vi "ARC_Queue Valid.vi"(8 "error in (no error)":errorcluster caption="Error In (no error)", 11 "Queue Name(unamed)":string) -> (0 "error out":errorcluster caption="Error Out", 2 "Not Exist?":bool, 3 "Empty Queue Name?":bool)   [LabVIEW 2016]
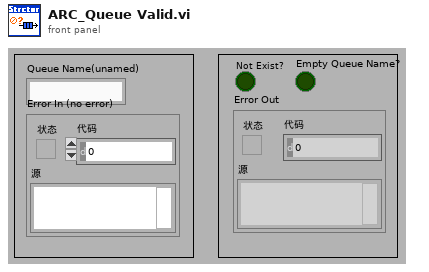
[diagram p1: front panel]
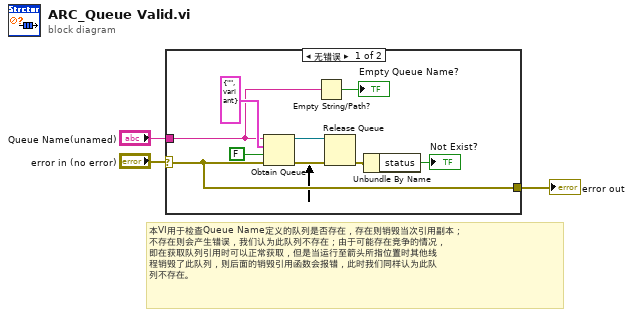
[diagram p0: block diagram]
diagram:
  # "本VI用于检查Queue Name定义的队列是否存在，存在则销毁当次引用副本；\n不存在则会产生错误，我们认为此队列不存在；由于可能存在竞争的情况，\n即在获取队列引用时可以正常获取，但是当运行至箭头所指位置时其他线\n程销毁了此队列，则后面的销毁引用函数会报错，此时我们同样认为此队\n列不存在。"
  n1 = case shown="无错误" "error in (no error)" {
    selector: "error in (no error)" -> [w11 w13]
    tunnel: [w11 w13] -> w2
    tunnel: "Queue Name(unamed)" -> [w5 _]
    frame No Error {
      n2 = Obtain Queue(name (unnamed)=w5, element data type=cluster{"Event":string, "Data":variant} {"Event"="", "Data"=variant} ("输出簇"), create if not found? (T)=FALSE ("如未找到是否创建？(T)"), error in (no error)=w11) -> (queue out=w9:refnum<queue>, error out=w10:errorcluster)  [unwired: 1 in, 1 out]
      n3 = Empty String/Path?(string/path=w5) -> (empty?=→"Empty Queue Name?":bool)
      n4 = Release Queue(queue=w9, error in (no error)=w10) -> (error out=w8:errorcluster)  [unwired: 1 in, 2 out]
      n5 = Unbundle By Name(w8) -> ("status"=→"Not Exist?":bool)
    }
    frame Error {
    }
  }
  "error out" <- w2
